vi "Clear CCD.vi"(8 "error in (no error)":errorcluster, 11 "CCDCamera in":refnum<class "CCDCamera.lvclass">) -> (0 "error out":errorcluster, 3 "CCDCamera out":refnum<class "CCDCamera.lvclass">)   [LabVIEW 2018, in "CCDCamera.lvclass"]
doc: "This VI acquire a bias image to clean the CCD."
uses:
  CCDCamera.lvclass
  CCDCamera.lvclass/CCDCamera.ctl
panel:
  out "Cluster":T1
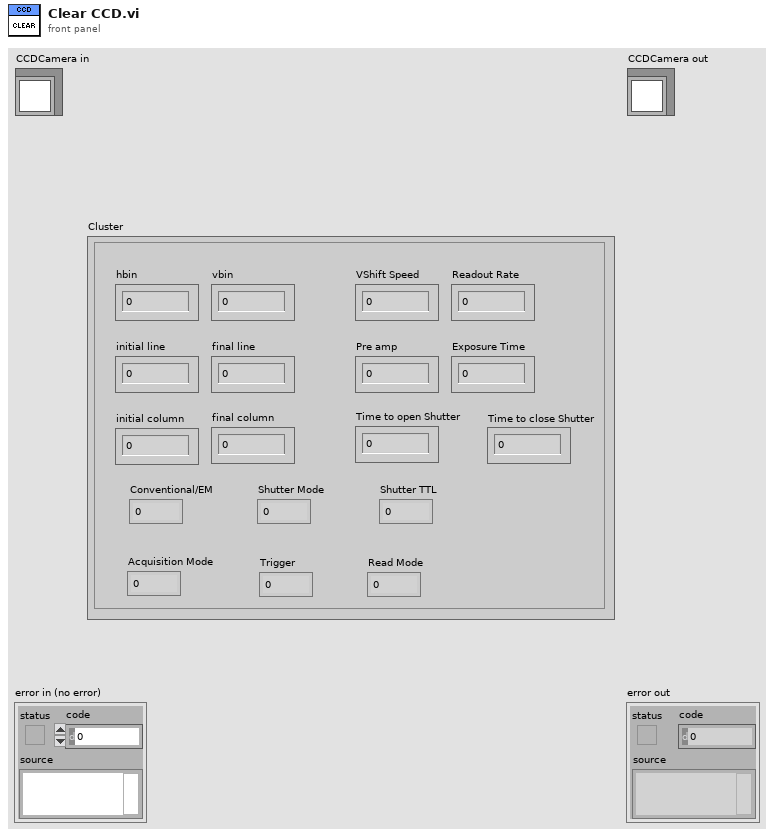
[diagram p1: front panel]
types:
  T1 = cluster{"hbin":dbl, "vbin":dbl, "initial line":dbl, "final line":dbl, "initial column":dbl, "final column":dbl, "VShift Speed":dbl, "Readout Rate":dbl, "Pre amp":dbl, "Exposure Time":dbl, "Conventional/EM":u16, "Shutter Mode":u16, "Shutter TTL":u16, "Trigger":u16, "Time to open Shutter":dbl, "Time to close Shutter":dbl, "Acquisition Mode":u16, "Read Mode":u16}
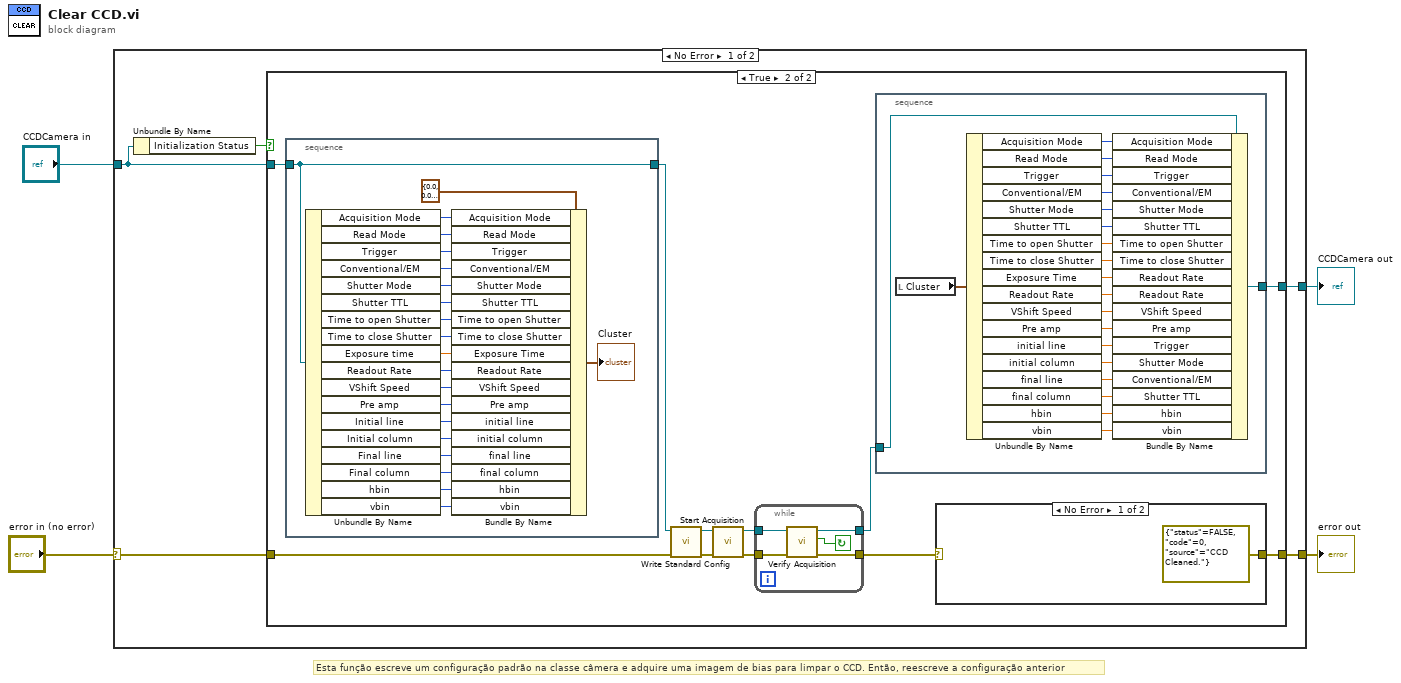
[diagram p0: block diagram]
diagram:
  # "Esta função escreve um configuração padrão na classe câmera e adquire uma imagem de bias para limpar o CCD. Então, reescreve a configuração anterior"
  n1 = case shown="No Error" "error in (no error)" {
    selector: "error in (no error)" -> [w9 w73]
    tunnel: "CCDCamera in" -> [w6 w72]
    tunnel: [w8 w72] -> w2
    tunnel: [w7 w73] -> w1
    frame No Error {
      n2 = Unbundle By Name(w6) -> ("Initialization Status"=w5:bool)
      n3 = case shown="True" w5 {
        tunnel: w6 -> [w10 w22]
        tunnel: w9 -> [w11 w17]
        tunnel: [w10 w13] -> w8
        tunnel: [w11 w12] -> w7
        frame False {
        }
        frame True {
          n4 = stacked-sequence {
            tunnel: w22 -> [w51]
            tunnel: [w51] -> w21
            frame #0 {
              n5 = Unbundle By Name(w51) -> ("Acquisition Mode"=w69:u16, "Read Mode"=w68:u16, "Trigger"=w67:u16, "Conventional/EM"=w66:u16, "Shutter Mode"=w65:u16, "Shutter TTL"=w64:u16, "Time to open Shutter"=w63:u16, "Time to close Shutter"=w62:u16, "Exposure time"=w61:dbl, "Readout Rate"=w60:u16, "VShift Speed"=w59:u16, "Pre amp"=w58:u16, "Initial line"=w57:u16, "Initial column"=w56:u16, "Final line"=w55:u32, "Final column"=w54:u32, "hbin"=w53:u16, "vbin"=w52:u16)
              n6 = Bundle By Name(cluster=T1 {"hbin"=0.0, "vbin"=0.0, "initial line"=0.0, "final line"=0.0, "initial column"=0.0, "final column"=0.0, "VShift Speed"=0.0, "Readout Rate"=0.0, "Pre amp"=0.0, "Exposure Time"=0.0, "Conventional/EM"=0, "Shutter Mode"=0, "Shutter TTL"=0, "Trigger"=0, "Time to open Shutter"=0.0, "Time to close Shutter"=0.0, "Acquisition Mode"=0, "Read Mode"=0} ("Cluster 2"), "Acquisition Mode"=w69, "Read Mode"=w68, "Trigger"=w67, "Conventional/EM"=w66, "Shutter Mode"=w65, "Shutter TTL"=w64, "Time to open Shutter"=w63, "Time to close Shutter"=w62, "Exposure Time"=w61, "Readout Rate"=w60, "VShift Speed"=w59, "Pre amp"=w58, "initial line"=w57, "initial column"=w56, "final line"=w55, "final column"=w54, "hbin"=w53, "vbin"=w52) -> (→"Cluster":T1)
            }
          }
          n7 = call "Write Standard Config.vi"("error in (no error)"=w17, "CCDCamera in"=w21) -> ("error out"=w16:errorcluster, "CCDCamera out"=w20:refnum<class "CCDCamera.lvclass">)  [unwired: 8 in]
          n8 = call "Start Acquisition.vi"("error in (no error)"=w16, "CCDCamera in"=w20) -> ("error out"=w15:errorcluster, "CCDCamera out"=w19:refnum<class "CCDCamera.lvclass">)  [unwired: 8 in]
          n9 = while {
            tunnel: w19 -> [w50]
            tunnel: [w48] -> w18
            tunnel: w15 -> [w47]
            tunnel: [w46] -> w14
            stop <- w49 continue-if-true
            n10 = call "Verify Acquisition.vi"("error in (no error)"=w47, "CCDCamera in"=w50) -> ("error out"=w48:errorcluster, "Acquiring"=w49:bool, "CCDCamera out"=w46:refnum<class "CCDCamera.lvclass">)  [unwired: 7 in]
          }
          n11 = stacked-sequence {
            tunnel: w14 -> [w25]
            tunnel: [w24] -> w13
            frame #0 {
              n12 = local read "Cluster"() -> (w23:T1)
              n13 = Unbundle By Name(w23) -> ("Acquisition Mode"=w43:u16, "Read Mode"=w42:u16, "Trigger"=w41:u16, "Conventional/EM"=w40:u16, "Shutter Mode"=w39:u16, "Shutter TTL"=w38:u16, "Time to open Shutter"=w37:dbl, "Time to close Shutter"=w36:dbl, "Exposure Time"=w35:dbl, "Readout Rate"=w34:dbl, "VShift Speed"=w33:dbl, "Pre amp"=w32:dbl, "initial line"=w31:dbl, "initial column"=w30:dbl, "final line"=w29:dbl, "final column"=w28:dbl, "hbin"=w27:dbl, "vbin"=w26:dbl)
              n14 = Bundle By Name(cluster=w25, "Acquisition Mode"=w43, "Read Mode"=w42, "Trigger"=w41, "Conventional/EM"=w40, "Shutter Mode"=w39, "Shutter TTL"=w38, "Time to open Shutter"=w37, "Time to close Shutter"=w36, "Readout Rate"=w35, "Readout Rate"=w34, "VShift Speed"=w33, "Pre amp"=w32, "Trigger"=w31, "Shutter Mode"=w30, "Conventional/EM"=w29, "Shutter TTL"=w28, "hbin"=w27, "vbin"=w26) -> (w24:refnum<class "CCDCamera.lvclass">)
            }
          }
          n15 = case shown="No Error" w18 {
            selector: w18 -> [_ w45]
            tunnel: [errorcluster {"status"=FALSE, "code"=0, "source"="CCD Cleaned."} ("error IO") w45] -> w12
            frame No Error {
            }
            frame Error {
            }
          }
        }
      }
    }
    frame Error {
    }
  }
  "error out" <- w1
  "CCDCamera out" <- w2
